vi "Offset by Size.vi"(8 "error in (no error)":errorcluster caption="错误输入（无错误）", 10 "Size.lvclass":refnum<class "Size.lvclass">, 11 "Point 输入":refnum<class "Point.lvclass"> caption="DNL_LabVIEW Object in") -> (0 "error out":errorcluster caption="错误输出", 3 "Point 输出":refnum<class "Point.lvclass"> caption="DNL_LabVIEW Object out")   [LabVIEW 2011, in "Point.lvclass"]
uses:
  Point.lvclass
  Size/Size.lvclass
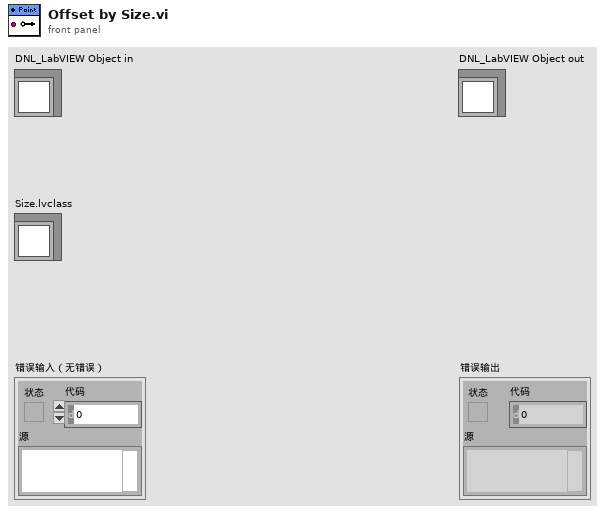
[diagram p1: front panel]
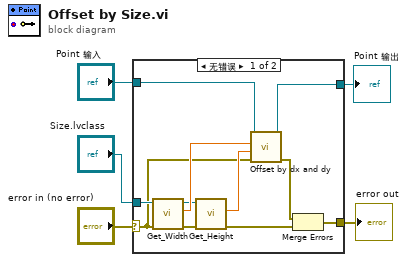
[diagram p0: block diagram]
diagram:
  n1 = case shown="无错误" "error in (no error)" {
    selector: "error in (no error)" -> [w10 w18]
    tunnel: [w7 w18] -> w4
    tunnel: [w6 w17] -> w2
    tunnel: "Point 输入" -> [w15 w17]
    tunnel: "Size.lvclass" -> [w16 _]
    frame No Error {
      n2 = call "Get_Width.vi"("error in (no error)"=w10, "Size输入"=w16) -> ("error out"=w12:errorcluster, "Width"=w14:dbl, "Size输出"=w13:refnum<class "Size.lvclass">)  [unwired: 7 in]
      n3 = call "Get_Height.vi"("error in (no error)"=w12, "Size输入"=w13) -> ("error out"=w8:errorcluster, "Height"=w11:dbl)  [unwired: 7 in, 1 out]
      n4 = call "Offset by dx and dy.vi"("error in (no error)"=w10, "dy"=w11, "dx"=w14, "Point 输入"=w15) -> ("error out"=w9:errorcluster, "Point 输出"=w6:refnum<class "Point.lvclass">)  [unwired: 6 in]
      n5 = Merge Errors(w9, w8) -> (w7:errorcluster)
    }
    frame Error {
    }
  }
  "error out" <- w4
  "Point 输出" <- w2
